vi "DataRefNew.vi"(8 "error in (no error)":errorcluster caption="错误输入（无错误）", 11 "MainPage 输入":refnum<class "MainPage.lvclass">) -> (0 "error out":errorcluster caption="错误输出", 2 "数据记录引用":refnum<data-value>, 3 "MainPage 输出":refnum<class "MainPage.lvclass">)   [LabVIEW 2019, in "MainPage.lvlib" / "MainPage.lvclass"]
uses:
  MainPage.lvclass
  MainPage.lvclass/MainPage.ctl
panel:
  in  "通讯接口记录":T1
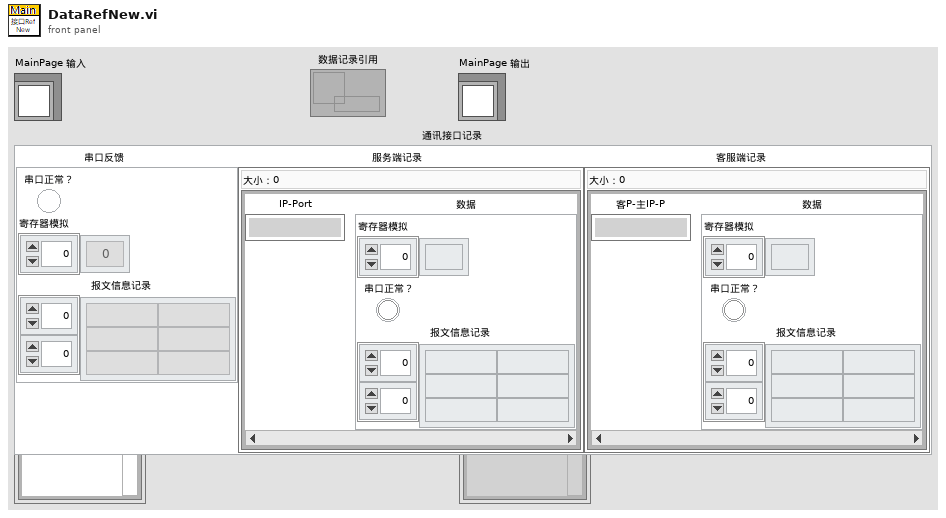
[diagram p1: front panel]
types:
  T1 = typedef "MainPage.lvlib/MainPage.lvclass/DataRef_通讯接口数据记录.ctl" = cluster{"串口反馈":cluster{"串口正常？":bool, "寄存器模拟":dbl[], "报文信息记录":string[][]}, "服务端记录":map{string, cluster{"寄存器模拟":dbl[], "串口正常？":bool, "报文信息记录":string[][]}}, "客服端记录":map{string, cluster{"寄存器模拟":dbl[], "串口正常？":bool, "报文信息记录":string[][]}}}
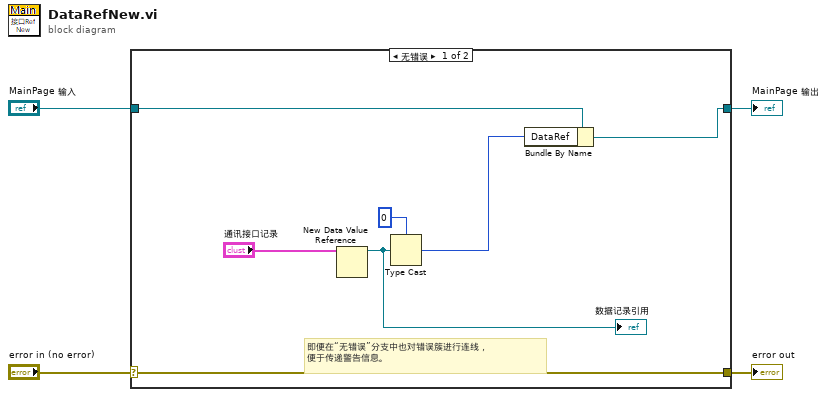
[diagram p0: block diagram]
diagram:
  n1 = case shown="无错误" "error in (no error)" {
    selector: "error in (no error)" -> [w11 w13]
    tunnel: [w11 w13] -> w3
    tunnel: [w5 w12] -> w1
    tunnel: "MainPage 输入" -> [w8 w12]
    frame No Error {
      # "即便在“无错误”分支中也对错误簇进行连线，\n便于传递警告信息。"
      n2 = New Data Value Reference(data value="通讯接口记录") -> (data value reference=w6:refnum<data-value>)  [unwired: 1 in, 1 out]
      "数据记录引用" <- w6
      n3 = Type Cast(type=u32 0 ("DataRef"), x=w6) -> (*(type *) &x=w7:u32)
      n4 = Bundle By Name(cluster=w8, "DataRef"=w7) -> (w5:refnum<class "MainPage.lvclass">)
    }
    frame Error {
    }
  }
  "error out" <- w3
  "MainPage 输出" <- w1
